vi "debugReadWrite.vi"() -> ()   [LabVIEW 2015, in "labOpenShowVar.lvlib"]
uses:
  <vilib>/Platform/TimedLoop/XDataNode/timing_clust.ctl
  <vilib>/Platform/TimedLoop/XDataNode/nitl_modes.ctl
  <vilib>/Platform/TimedLoop/XDataNode/wakeup.ctl
  <vilib>/Platform/TimedLoop/XDataNode/XDataNode.xnode
  labOpenShowVar.lvlib
  <vilib>/Platform/TimedLoop/XDataNode/XDNodeRunTimeDep.lvlib
panel:
  in  "写入":bool
  in  "writeData":string
  out "无符号字节数组":u8[](array[numeric])
  out "长度":i16
  out "data":string
  in  "cmd":string="aaa"
  in  "停止":bool
  in  "地址":string="172.31.1.147"
  # "简单的变量读写"
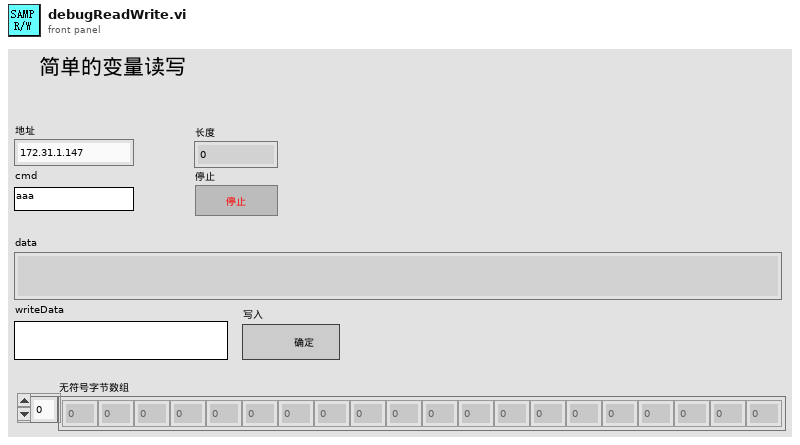
[diagram p1: front panel]
types:
  T1 = typedef "XDNodeRunTimeDep.lvlib/timing_clust.ctl" = cluster{"Expected End [f-1]":u64, "Actual End [f-1]":u64, "Finished Late? [f-1]":bool, "Expected End [i-1]":u64, "Actual End [i-1]":u64, "Finished Late? [i-1]":bool, "Expected Start [i]":u64, "Actual Start [i]":u64, "Expected Start [f]":u64, "Actual Start [f]":u64, "Source Name":string, "Structure Name":string, "Period":i64, "Deadline":i64, "Offset":i64, "Start":i64, "Priority":i32, "Timeout":i32, "Mode":T2, "Wakeup Reason":T3, "Error":errorcluster, "Source Type":string, "Secondary Source Type":string, "Global End Time":u64, "Global Start Time":u64, "Frame Duration":u64, "Iteration Duration":u64, "Assigned CPU":i32, "I/O Scan Engine Mode":u32}
  T2 = typedef "XDNodeRunTimeDep.lvlib/nitl_modes.ctl" = enum32{"No Change", "Process missed periods, maintain original phase", "Discard missed periods, maintain original phase", "Process missed periods, ignore original phase", "Discard missed periods, ignore original phase"}
  T3 = typedef "XDNodeRunTimeDep.lvlib/wakeup.ctl" = enum32{"Normal", "Aborted", "Asynchronous wakeup", "Timing source error", "Timed loop error", "Timeout"}
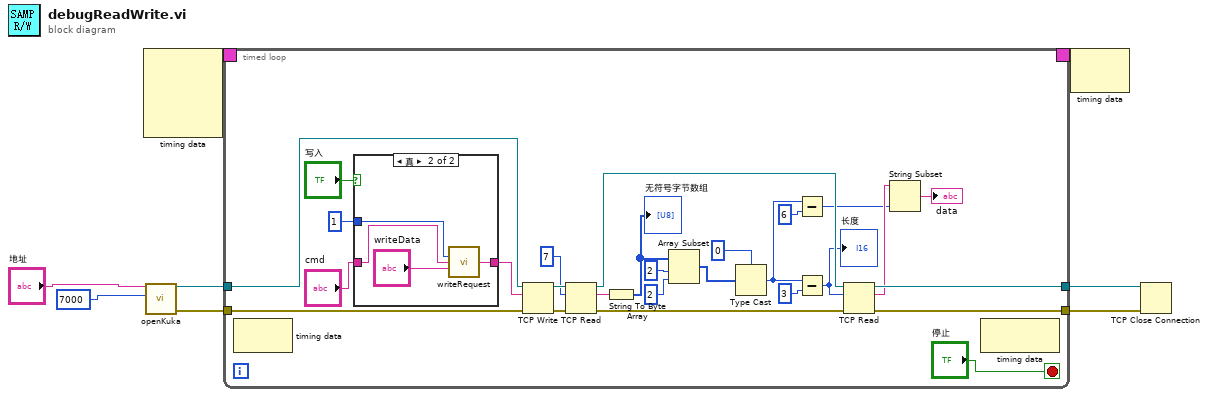
[diagram p0: block diagram]
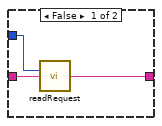
[diagram p2: hidden frame]
diagram:
  n1 = node-c288() -> (w4:T1)  [unwired: 4 in]
  n2 = call "openKuka.vi"("远程端口或服务名称"=u16 7000, "地址"="地址") -> ("错误输出"=w5:errorcluster, "TCP网络连接输出"=w6:refnum<k5>)  [unwired: 8 in]
  n3 = timed-loop {
    tunnel: w6 -> [w34]
    tunnel: w5 -> [w30]
    tunnel: [w19] -> w1
    tunnel: [w18] -> w2
    timing: w4 -> [_]
    timing-out: [_] -> w3
    stop <- "停止" stop-if-true
    n4 = node-c288() -> ()  [unwired: 1 in, 1 out]
    n5 = case shown="真" "写入" {
      tunnel: u16 1 ("id") -> [w38 w42]
      tunnel: "cmd" -> [w37 w41]
      tunnel: [w36 w40] -> w31
      frame False {
        n6 = call "readRequest.vi"("id"=w38, "cmd"=w37) -> ("readRequest"=w36:string)  [unwired: 13 in]
      }
      frame True {
        n7 = call "writeRequest.vi"("id"=w42, "cmd"=w41, "data"="writeData") -> ("readRequest"=w40:string)  [unwired: 12 in]
      }
    }
    n8 = TCP Write(connection ID=w34, data in=w31, error in (no error)=w30) -> (connection ID out=w29:refnum<k5>, error out=w28:errorcluster)  [unwired: 1 in, 1 out]
    n9 = TCP Read(connection ID=w29, bytes to read=7 ("读取的字节"), error in (no error)=w28) -> (connection ID out=w21:refnum<k5>, data out=w26:string, error out=w20:errorcluster)  [unwired: 2 in]
    n10 = String To Byte Array(string=w26) -> (unsigned byte array=w17:u8[])
    "无符号字节数组" <- w17
    n11 = Array Subset(array=w17, index=2 ("索引"), length=2 ("长度")) -> (w23:u8[])
    n12 = Type Cast(type=i16 0, x=w23) -> (*(type *) &x=w11:i16)
    n13 = Subtract(x=w11, y=i16 6) -> (x-y=w13:i16)
    n14 = Subtract(x=w11, y=i16 3) -> (x-y=w16:i16)
    "长度" <- w16
    n15 = TCP Read(connection ID=w21, bytes to read=w16, error in (no error)=w20) -> (connection ID out=w18:refnum<k5>, data out=w15:string, error out=w19:errorcluster)  [unwired: 2 in]
    n16 = String Subset(string=w15, length (rest)=w13) -> (substring=→"data":string)  [unwired: 1 in]
    n17 = node-c288() -> ()  [unwired: 1 in, 1 out]
  }
  n18 = node-c288(w3) -> ()  [unwired: 1 out]
  n19 = TCP Close Connection(connection ID=w2, error in (no error)=w1) -> ()  [unwired: 1 in, 2 out]
